vi "Run.vi"(8 "error in (no error)":errorcluster, 11 "AF MQTT Message Channel in":refnum<class "AF MQTT Message Channel.lvclass">) -> (0 "error out":errorcluster, 3 "AF MQTT Message Channel out":refnum<class "AF MQTT Message Channel.lvclass">)   [LabVIEW 2020, in "AF MQTT Channel.lvlib" / "AF MQTT Message Channel.lvclass"]
uses:
  AF MQTT Message Channel.lvclass
  C:/Users/Simon/Documents/GitHub/LV-Actor-Pub-Sub/Source/Actor Pub Sub Channels/Pub Sub Message Channel/Pub Sub Message Channel.lvclass
  AF MQTT Message Channel.lvclass/AF MQTT Message Channel.ctl
  <vilib>/LabVIEW Open Source Project/MQTT Client/Client class/Client.lvclass/Client.ctl
  <vilib>/ActorFramework/Message Dequeuer/Dequeue Priority.ctl
  <vilib>/ActorFramework/Message/Message.lvclass
  c3a9c27e-0f89-4d5a-88dd-89df27bcec45.vi
  <vilib>/LabVIEW Open Source Project/MQTT Client/Client class/Client.lvclass
  C:/Program Files (x86)/National Instruments/LabVIEW 2020/vi.lib/LabVIEW Open Source Project/MQTT Connection/MQTT_Base/Base Class/MQTT_Base.lvclass
  Actor Pub Sub Channels/Pub Sub Message Channel/Pub Sub Message Channel.lvclass
  <vilib>/LabVIEW Open Source Project/MQTT Control Packets/Control Packets/PUBLISH/PUBLISH.lvclass
  <vilib>/regexp/Match Regular Expression.xnode
  <vilib>/LabVIEW Open Source Project/MQTT Connection/MQTT_Base/Base Class/MQTT_Base.lvclass
  <vilib>/ActorFramework/Message Dequeuer/Message Dequeuer.lvclass
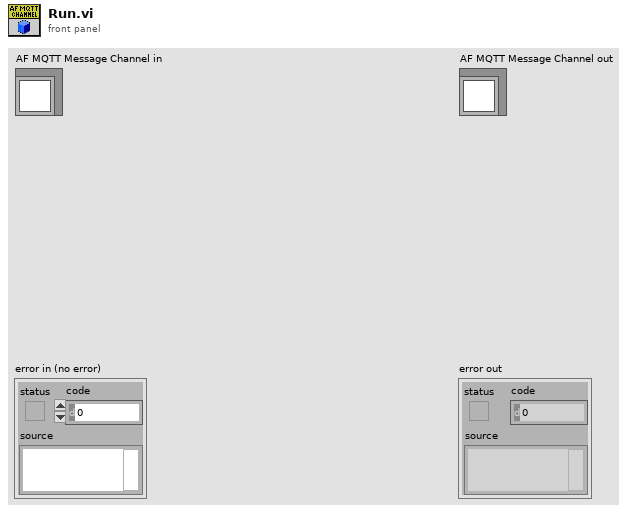
[diagram p1: front panel]
types:
  T1 = typedef "MQTT Client.lvlib/Client.lvclass/Public Events -- cluster.ctl" = cluster{"Connection Status":refnum<user-event>, "Connected":refnum<user-event>, "Application Message":refnum<user-event>}
  T2 = typedef "Actor Framework.lvlib/Message Dequeuer.lvclass/Dequeue Priority.ctl" = enum16{"Low", "Normal", "High", "Critical"}
  T3 = typedef "MQTT_Control_Packets.lvlib/CONNECT.lvclass/ConnectFlags -- cluster.ctl" = cluster{"Reserved":bool, "Clean Session":bool, "Will Flag":bool, "Will QoS 1":bool, "Will QoS 2":bool, "Will Retain":bool, "Password Flag":bool, "User Name Flag":bool}
  T4 = cluster{"Will Topic":string, "Will Message":string, "Username":string, "Password":string}
  T5 = typedef "MQTT_Control_Packets.lvlib/ControlPacket.lvclass/QualityOfService -- enum.ctl" = enum16{"0 (At Most Once)", "1 (At Least Once)", "2 (Exactly Once)"}
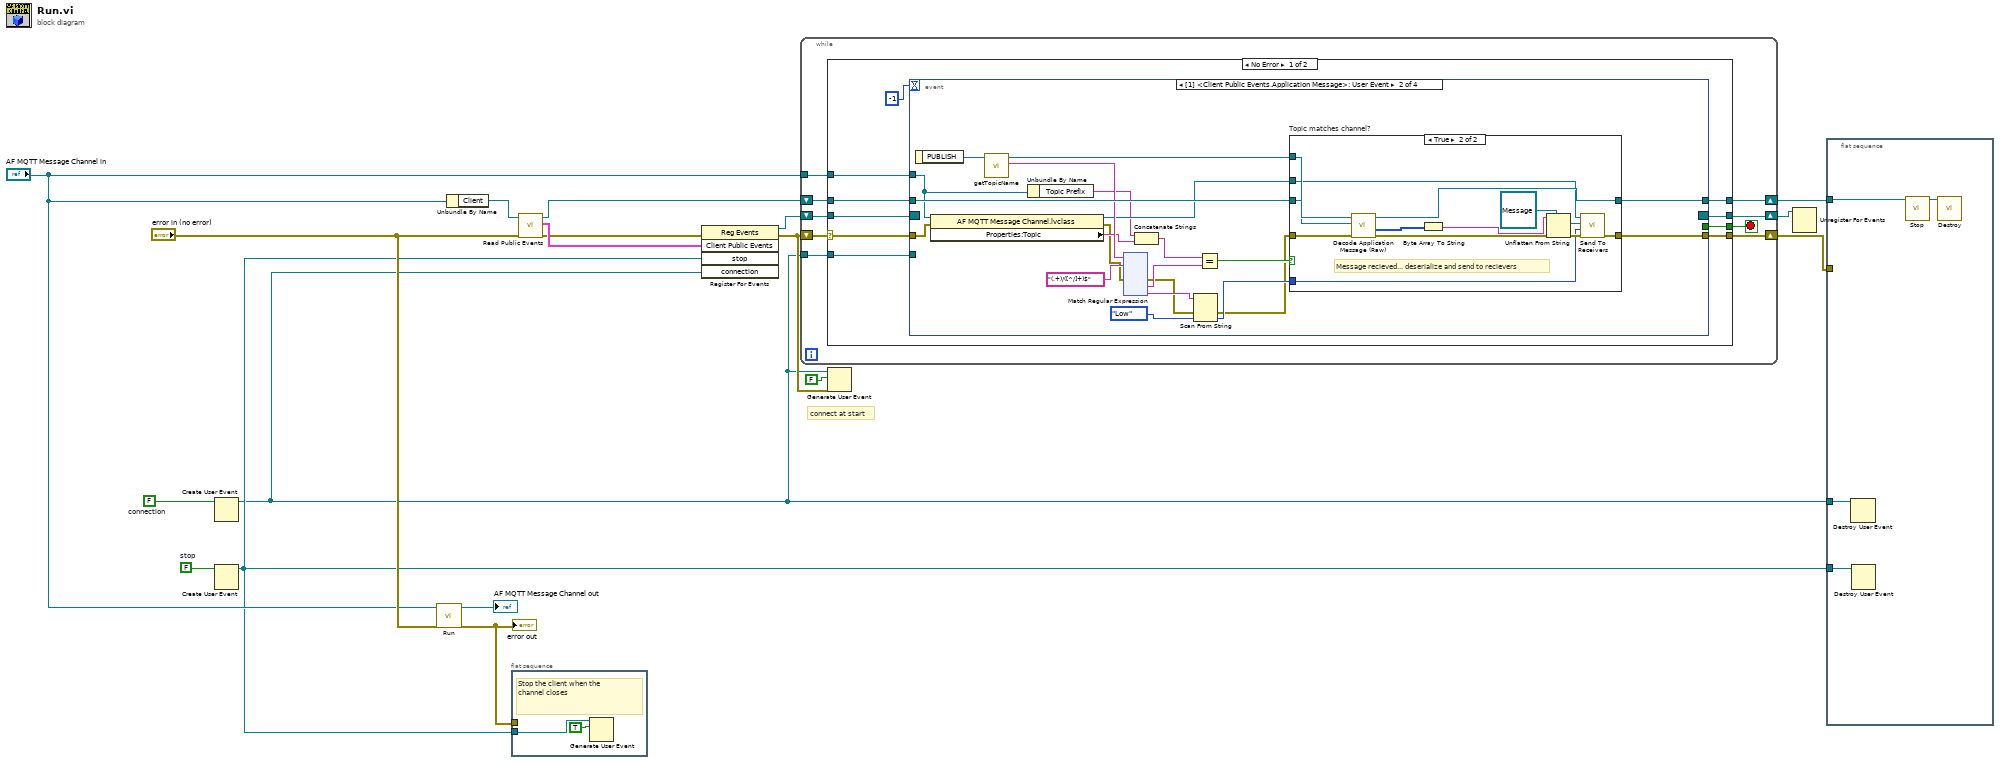
[diagram p0: block diagram]
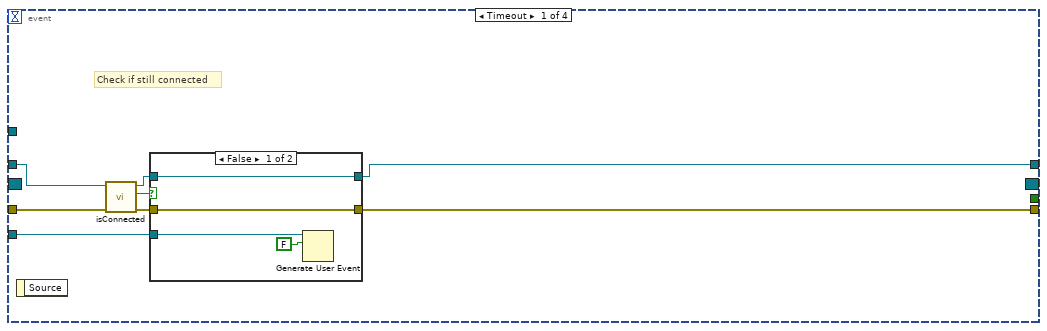
[diagram p2: hidden frame]
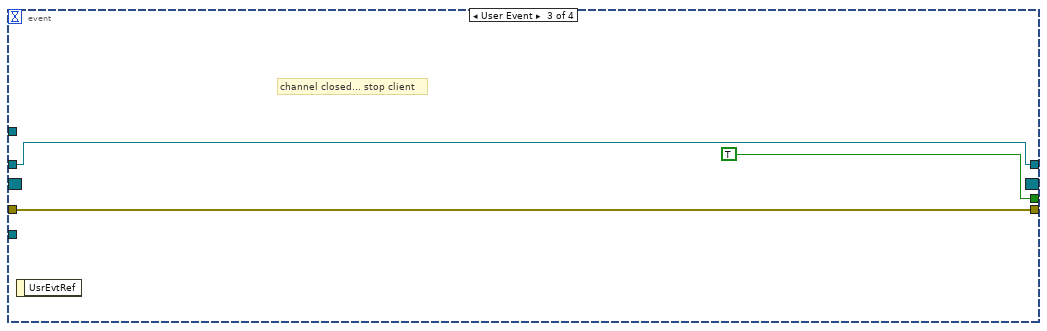
[diagram p5: hidden frame]
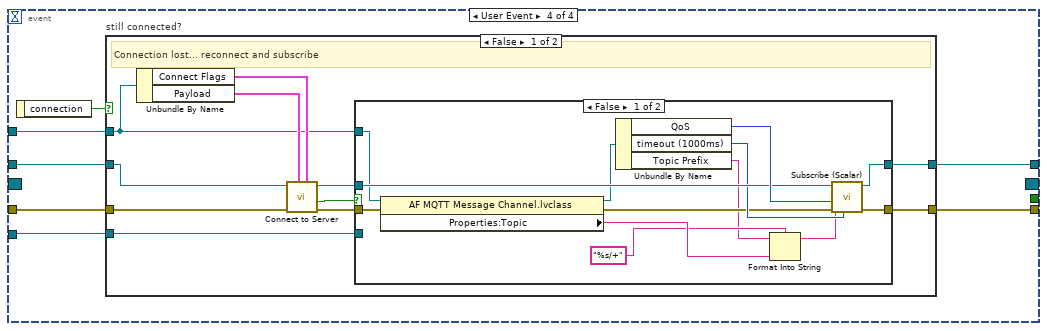
[diagram p6: hidden frame]
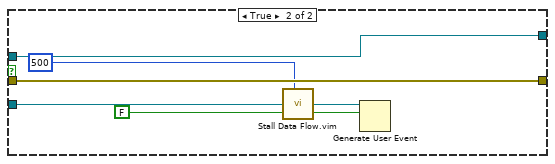
[diagram p7: hidden frame]
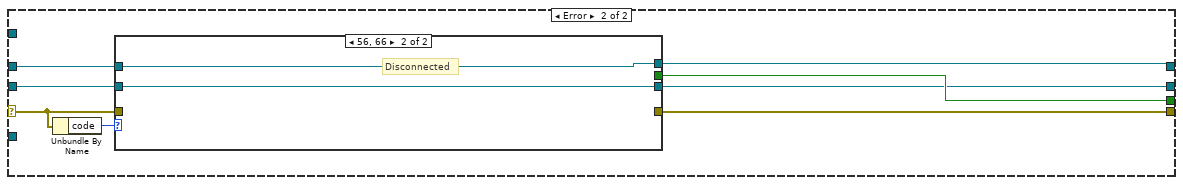
[diagram p9: hidden frame]
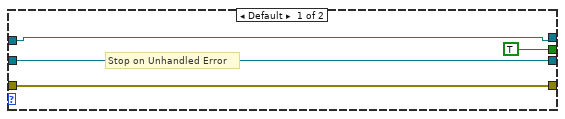
[diagram p10: hidden frame]
diagram:
  w7 = FALSE  # connection
  w9 = FALSE  # stop
  # "connect at start"
  n1 = Create User Event(user event datatype=w7) -> (user event=w4:refnum<user-event>)  [unwired: 1 in, 1 out]
  n2 = Create User Event(user event datatype=w9) -> (user event=w6:refnum<user-event>)  [unwired: 1 in, 1 out]
  n3 = call-parent "Run.vi"("error in (no error)"="error in (no error)", "Pub Sub Message Channel in"="AF MQTT Message Channel in") -> ("error out"=w8:errorcluster, "Pub Sub Message Channel out"=→"AF MQTT Message Channel out":refnum<class "AF MQTT Message Channel.lvclass">)  [unwired: 8 in]
  "error out" <- w8
  n4 = Unbundle By Name("AF MQTT Message Channel in") -> ("Client"=w12:refnum<class "Client.lvclass">)
  n5 = flat-sequence {
    tunnel: w8 -> [_]
    tunnel: w6 -> [w20]
    frame #0 {
      # "Stop the client when the channel closes"
      n6 = Generate User Event(user event=w20, event data cluster=TRUE ("event data")) -> ()  [unwired: 2 in, 2 out]
    }
  }
  n7 = call <vilib>:"Read Public Events.vi"("error in (no error)"="error in (no error)", "Client in"=w12) -> ("error out"=w14:errorcluster, "Client Public Events"=w15:T1, "Client out"=w13:refnum<class "Client.lvclass">)  [unwired: 7 in]
  n8 = register-events(error in=w14, w15, w6, w4) -> (reference out=w16:refnum<event-registration>, error out=w5:errorcluster)  [unwired: 1 in]
  n9 = while {
    shift-right: [w28] -> w17
    shift-left: w16 -> [w29]
    shift-right: [w25] -> w1
    shift-left: w13 -> [w26]
    shift-right: [w27] -> w2
    shift-left: w5 -> [w23]
    tunnel: "AF MQTT Message Channel in" -> [w22]
    tunnel: w4 -> [w21]
    stop <- w24 stop-if-true
    n10 = case shown="No Error" w23 {
      selector: w23 -> [w32 w251]
      tunnel: w29 -> [w39 w250]
      tunnel: [w38 w249] -> w28
      tunnel: [w37 w253] -> w27
      tunnel: w26 -> [w35 w254]
      tunnel: [w34 w256] -> w25
      tunnel: [w33 w252] -> w24
      tunnel: w22 -> [w31 _]
      tunnel: w21 -> [w30 _]
      frame No Error {
        n11 = event shown="[1] <Client Public Events.Application Message>: User Event" {
          selector: w39 -> [_ _ _ _]
          dyn-events: [_ _ _ _] -> w38
          timeout: -1 -> [_ _ _ _]
          tunnel: w32 -> [w43 w71 w208 w212]
          tunnel: [w46 w69 w208 w213] -> w37
          tunnel: [_ _ TRUE _] -> w33
          tunnel: w35 -> [w45 w72 w209 w216]
          tunnel: [w47 w70 w209 w214] -> w34
          tunnel: w31 -> [_ w60 _ w211]
          tunnel: w30 -> [w40 _ _ w210]
          event Timeout {
            # "Check if still connected"
            n12 = event-data() -> ()  [unwired: 1 in, 1 out]
            n13 = call <vilib>:"isConnected.vi"("error in (no error)"=w43, "Client in"=w45) -> ("error out"=w42:errorcluster, "connected"=w41:bool, "Client out"=w44:refnum<class "Client.lvclass">)  [unwired: 7 in]
            n14 = case shown="False" w41 {
              tunnel: [w51 w53] -> w47
              tunnel: [w50 w52] -> w46
              tunnel: w44 -> [w51 w53]
              tunnel: w42 -> [w50 w52]
              tunnel: w40 -> [w49 _]
              frame False {
                n15 = Generate User Event(user event=w49, event data cluster=FALSE ("Connection")) -> ()  [unwired: 2 in, 2 out]
              }
              frame True {
              }
            }
          }
          event User Event {
            n16 = event-data() -> ("PUBLISH"=w74:refnum<class "PUBLISH.lvclass">)  [unwired: 1 in]
            n17 = property class="AF MQTT Message Channel.lvclass"(reference=w60, error in=w71) -> (reference out=w61:refnum<class "AF MQTT Message Channel.lvclass">, error out=w55:errorcluster, "Properties:Topic"=w58:string)
            n18 = call <vilib>:"getTopicName.vi"("PUBLISH in"=w74) -> ("Topic"=w67:string, "PUBLISH out"=w73:refnum<class "PUBLISH.lvclass">)  [unwired: 8 in, 1 out]
            n19 = Unbundle By Name(w60) -> ("Topic Prefix"=w59:string)
            n20 = xnode "Match Regular Expression"("input string"=w67, "regular expression"="(.+)/([^/]+)$", "error in"=w55) -> ("error out"=w56:errorcluster, "submatch 1"=w65:string, "submatch 2"=w63:string)  [unwired: 3 in, 4 out]
            n21 = Concatenate Strings(w59, w58) -> (w57:string)
            n22 = Scan From String(input string=w63, error in=w56, default 1=Dequeue_Priority."Low" ("priority")) -> (error out=w54:errorcluster, output 1=w62:T2)  [unwired: 2 in, 2 out]
            n23 = Equal?(x=w57, y=w65) -> (x = y?=w68:bool)
            n24 = case "Topic matches channel?" shown="True" w68 {
              tunnel: w73 -> [_ w205]
              tunnel: w72 -> [w193 w206]
              tunnel: w54 -> [w192 w204]
              tunnel: [w193 w203] -> w70
              tunnel: [w192 w197] -> w69
              tunnel: w61 -> [_ w196]
              tunnel: w62 -> [_ w194]
              frame False {
              }
              frame True {
                # "Message recieved... deserialize and send to recievers"
                n25 = call <vilib>:"Decode Application Message (Raw).vi"("error in (no error)"=w204, "PUBLISH"=w205, "Client in"=w206) -> ("error out"=w199:errorcluster, "Payload"=w202:u8[], "Client out"=w203:refnum<class "Client.lvclass">)  [unwired: 5 in, 1 out]
                n26 = Byte Array To String(unsigned byte array=w202) -> (string=w201:string)
                n27 = Unflatten From String(type=refnum<class "Message.lvclass"> refnum ("Message"), binary string=w201, error in (no error)=w199) -> (value=w195:refnum<class "Message.lvclass">, error out=w198:errorcluster)  [unwired: 2 in, 1 out]
                n28 = call "Send To Receivers.vi"("error in (no error)"=w198, "priority"=w194, "Message"=w195, "Pub Sub Message Channel in"=w196) -> ("error out"=w197:errorcluster)  [unwired: 7 in]
              }
            }
          }
          event User Event {
            # "channel closed... stop client"
            n29 = event-data() -> ()  [unwired: 1 in, 1 out]
          }
          event User Event {
            n30 = event-data() -> ("connection"=w215:bool)  [unwired: 1 in]
            n31 = case "still connected?" shown="False" w215 {
              tunnel: w216 -> [w227 w247]
              tunnel: [w222 w247] -> w214
              tunnel: [w220 w248] -> w213
              tunnel: w212 -> [w226 w248]
              tunnel: w211 -> [w219 _]
              tunnel: w210 -> [w217 _]
              frame False {
                # "Connection lost... reconnect and subscribe"
                n32 = Unbundle By Name(w219) -> ("Connect Flags"=w225:T3, "Payload"=w224:T4)
                n33 = call <vilib>:"Connect to Server.vi"("Connect Flags"=w225, "Payload"=w224, "error in (no error)"=w226, "Client in"=w227) -> ("error out"=w221:errorcluster, "timed out"=w218:bool, "Client out"=w223:refnum<class "Client.lvclass">)  [unwired: 4 in, 1 out]
                n34 = case shown="False" w218 {
                  tunnel: w223 -> [w239 w246]
                  tunnel: [w238 w246] -> w222
                  tunnel: w221 -> [w237 w245]
                  tunnel: [w236 w245] -> w220
                  tunnel: w219 -> [w233 _]
                  tunnel: w217 -> [_ w244]
                  frame False {
                    n35 = property class="AF MQTT Message Channel.lvclass"(reference=w233, error in=w237) -> (reference out=w232:refnum<class "AF MQTT Message Channel.lvclass">, error out=w234:errorcluster, "Properties:Topic"=w231:string)
                    n36 = Unbundle By Name(w232) -> ("QoS"=w240:T5, "timeout (1000ms)"=w235:i32, "Topic Prefix"=w228:string)
                    n37 = Format Into String(format string="%s/+", initial string=w228, w231) -> (resulting string=w229:string)  [unwired: 1 in, 1 out]
                    n38 = call <vilib>:"Subscribe (Scalar).vi"("timeout (1000ms)"=w235, "error in (no error)"=w234, "QoS"=w240, "Topic Filter"=w229, "Client in"=w239) -> ("error out"=w236:errorcluster, "Client out"=w238:refnum<class "Client.lvclass">)  [unwired: 4 in, 1 out]
                  }
                  frame True {
                    n39 = call "Stall Data Flow.vim"("value in"=w244, "milliseconds to wait"=u32 500) -> ("value out"=w242:refnum<user-event>)  [unwired: 1 out]
                    n40 = Generate User Event(user event=w242, event data cluster=FALSE ("event data")) -> ()  [unwired: 2 in, 2 out]
                  }
                }
              }
              frame True {
              }
            }
          }
        }
      }
      frame Error {
        n41 = Unbundle By Name(w251) -> ("code"=w255:i32)
        n42 = case shown="56, 66" w255 {
          tunnel: w254 -> [w260 w262]
          tunnel: [w260 w262] -> w256
          tunnel: w251 -> [w259 _]
          tunnel: [w259 _] -> w253
          tunnel: [TRUE _] -> w252
          tunnel: w250 -> [w257 w261]
          tunnel: [w257 w261] -> w249
          frame Default {
            # "Stop on Unhandled Error"
          }
          frame 56, 66 {
            # "Disconnected"
          }
        }
      }
    }
  }
  n43 = Generate User Event(user event=w4, event data cluster=FALSE ("event data"), error in=w5) -> ()  [unwired: 1 in, 2 out]
  n44 = Unregister For Events(event registration refnum=w17) -> ()  [unwired: 1 in, 1 out]
  n45 = flat-sequence {
    tunnel: w2 -> [_]
    tunnel: w6 -> [w266]
    tunnel: w4 -> [w265]
    tunnel: w1 -> [w263]
    frame #0 {
      n46 = Destroy User Event(user event=w265) -> ()  [unwired: 1 in, 1 out]
      n47 = Destroy User Event(user event=w266) -> ()  [unwired: 1 in, 1 out]
      n48 = call <vilib>:"Stop.vi"("MQTT_Base in"=w263) -> ("MQTT_Base out"=w264:refnum<class "Client.lvclass">)  [unwired: 8 in, 2 out]
      n49 = call <vilib>:"Destroy.vi"("MQTT_Base in"=w264) -> ()  [unwired: 9 in, 2 out]
    }
  }
